vi "Load.vi"(5 "Autoshutdown? (T)":bool=TRUE, 7 "StartupParams":variant, 8 "error in (no error)":errorcluster, 11 "RQMHModule in":refnum<class "Module.lvclass">) -> (0 "error out":errorcluster, 3 "RQMHModule out":refnum<class "Module.lvclass">)   [LabVIEW 2024, in "Module.lvclass"]
uses:
  Module.lvclass
  Module.lvclass/Module.ctl
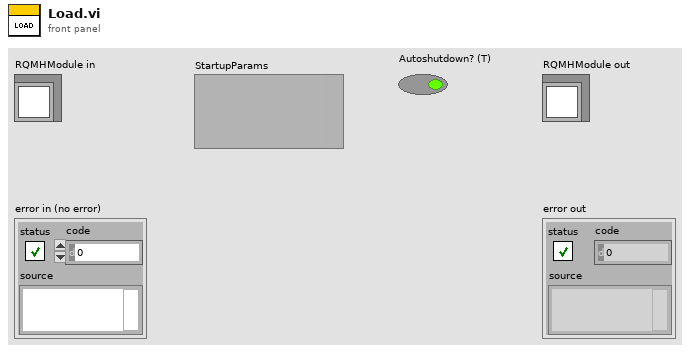
[diagram p1: front panel]
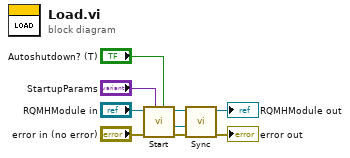
[diagram p0: block diagram]
diagram:
  n1 = call "Start.vi"("Autoshutdown? (T)"="Autoshutdown? (T)", "StartupParams"="StartupParams", "error in (no error)"="error in (no error)", "JQMHCore in"="RQMHModule in") -> ("error out"=w8:errorcluster, "StartupHandshake out"=w7:refnum<class "ModuleStartup.lvclass">, "JQMHCore out"=w9:refnum<class "Module.lvclass">)  [unwired: 5 in]
  n2 = call "Sync.vi"("error in (no error)"=w8, "StartupHandshake out"=w7, "JQMHCore in"=w9) -> ("error out"=→"error out":errorcluster, "JQMHCore out"=→"RQMHModule out":refnum<class "Module.lvclass">)  [unwired: 7 in]
